vi "From Serial Form.vi"(6 "Serial Version":T1, 10 "Deserializer in":refnum<class "Deserializer.lvclass">, 11 "PAS Data in":refnum<class "PAS Data.lvclass">) -> (0 "error out":errorcluster, 2 "Deserializer out":refnum<class "Deserializer.lvclass">, 3 "PAS Data out":refnum<class "PAS Data.lvclass">)   [LabVIEW 2014, in "PAS Data.lvclass"]
uses:
  PAS Data.lvclass
  <vilib>/NI/AQ Character Lineator/Deserializer/Deserializer.lvclass
  <vilib>/NI/AQ Character Lineator/Serialization Common/Serial Version.ctl
  Cell/PAS Cell Data.lvclass
  PAS Data.lvclass/PAS Data.ctl
  <vilib>/NI/AQ Character Lineator/Serializable/Remove Boolean.vi
  Data/Data.lvclass
  <vilib>/NI/AQ Character Lineator/Serializable/Serializable.lvclass
  <vilib>/NI/AQ Character Lineator/Serialization Common/Serialization Common.lvlib
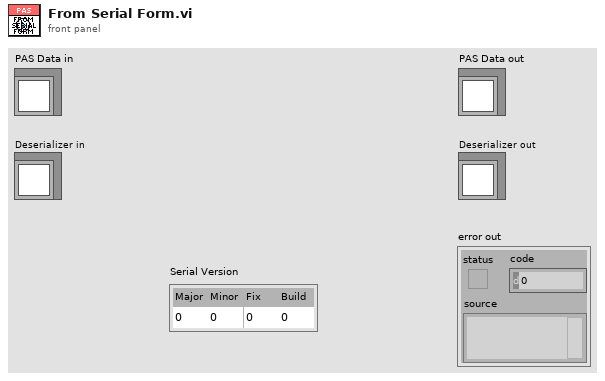
[diagram p1: front panel]
types:
  T1 = typedef "Serialization Common.lvlib/Serial Version.ctl" = cluster{"Major":u16, "Minor":u16, "Fix":u16, "Build":u16}
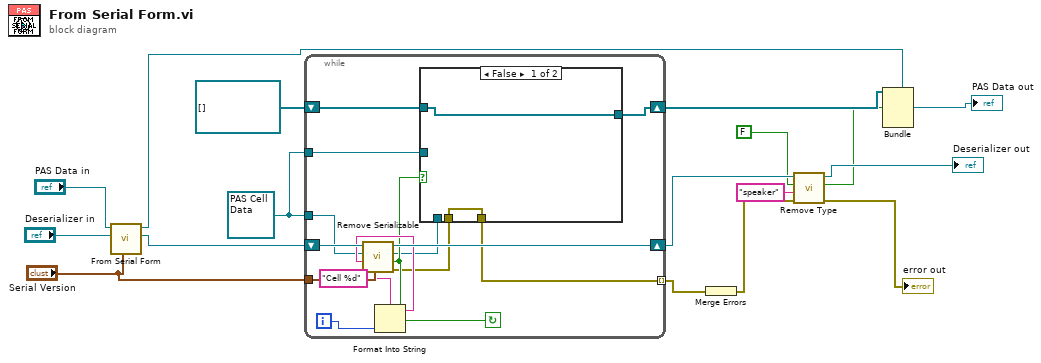
[diagram p0: block diagram]
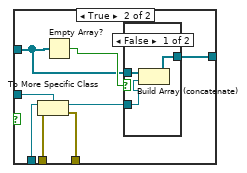
[diagram p2: hidden frame]
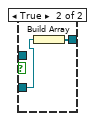
[diagram p3: hidden frame]
diagram:
  w13 = refnum<class "PAS Cell Data.lvclass"> refnum ("Cell Data")
  n1 = call-parent "From Serial Form.vi"("Serial Version"="Serial Version", "Deserializer in"="Deserializer in", "Data in"="PAS Data in") -> ("Deserializer out"=w15:refnum<class "Deserializer.lvclass">, "Data out"=w4:refnum<class "PAS Data.lvclass">)  [unwired: 6 in, 1 out]
  n2 = while {
    shift-right: [w30] -> w11
    shift-left: w15 -> [w31]
    tunnel: "Serial Version" -> [w29]
    tunnel: w13 -> [w25]
    tunnel: w13 -> [w23]
    shift-right: [w21] -> w3
    shift-left: refnum<class "PAS Cell Data.lvclass">[] [] -> [w22]
    tunnel: [w18] -> w10 mode=indexing
    i -> [w27]
    stop <- w24 continue-if-true
    n3 = Format Into String(format string="Cell %d", w27) -> (resulting string=w26:string)  [unwired: 2 in, 1 out]
    n4 = call <vilib>:"Remove Serializable.vi"("Serial Version"=w29, "Name"=w26, "Default Value"=w25, "Deserializer in"=w31) -> ("error out"=w19:errorcluster, "Found?"=w24:bool, "Serializable"=w20:refnum<class "Serializable.lvclass">, "Deserializer out"=w30:refnum<class "Deserializer.lvclass">)  [unwired: 4 in]
    n5 = case shown="False" w24 {
      tunnel: w23 -> [_ w41]
      tunnel: w22 -> [w33 w37]
      tunnel: [w33 w38] -> w21
      tunnel: w20 -> [_ w36]
      tunnel: w19 -> [w32 w35]
      tunnel: [w32 w34] -> w18
      frame False {
      }
      frame True {
        n6 = To More Specific Class(target class=w41, reference=w36, error in=w35) -> (specific class reference=w40:refnum<class "PAS Cell Data.lvclass">, error out=w34:errorcluster)
        n7 = Empty Array?(array=w37) -> (empty?=w39:bool)
        n8 = case shown="False" w39 {
          tunnel: w40 -> [w42 w46]
          tunnel: [w43 w45] -> w38
          tunnel: w37 -> [w44 _]
          frame False {
            n9 = Build Array (concatenate)(w44, w42) -> (w43:refnum<class "PAS Cell Data.lvclass">[])
          }
          frame True {
            n10 = Build Array(w46) -> (w45:refnum<class "PAS Cell Data.lvclass">[])
          }
        }
      }
    }
  }
  n11 = Merge Errors(w10) -> (w9:errorcluster)
  n12 = call-poly <vilib>:"Remove Type.vi"("error in (no error)"=w9, "Name"="speaker", "Default Value"=FALSE, "Deserializer in"=w11) -> ("error out"=→"error out":errorcluster, "Boolean"=w2:bool, "Deserializer out"=→"Deserializer out":refnum<class "Deserializer.lvclass">)  [unwired: 4 in, 1 out]
  n13 = Bundle(cluster=w4, w3, w2) -> (→"PAS Data out":refnum<class "PAS Data.lvclass">)  [unwired: 3 in]
